vi "bt_host_rule.vi"(11 "배열":sgl[](array[numeric])) -> (2 "Received":bool=TRUE, 3 "Correct?":bool)   [LabVIEW 2023]
panel:
  out "Raw Data":sgl[](array[numeric])
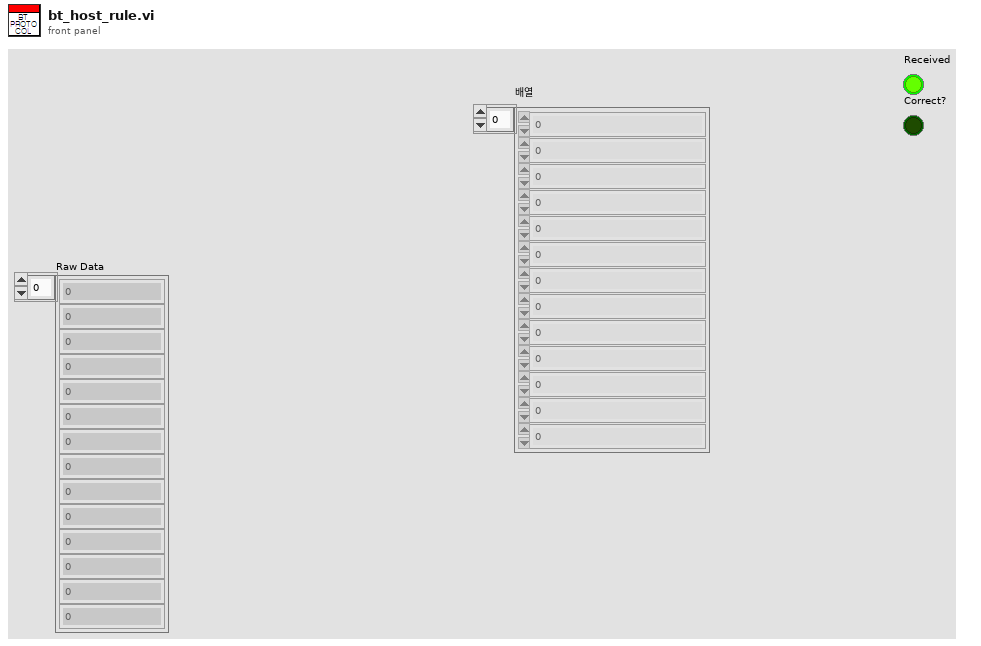
[diagram p1: front panel]
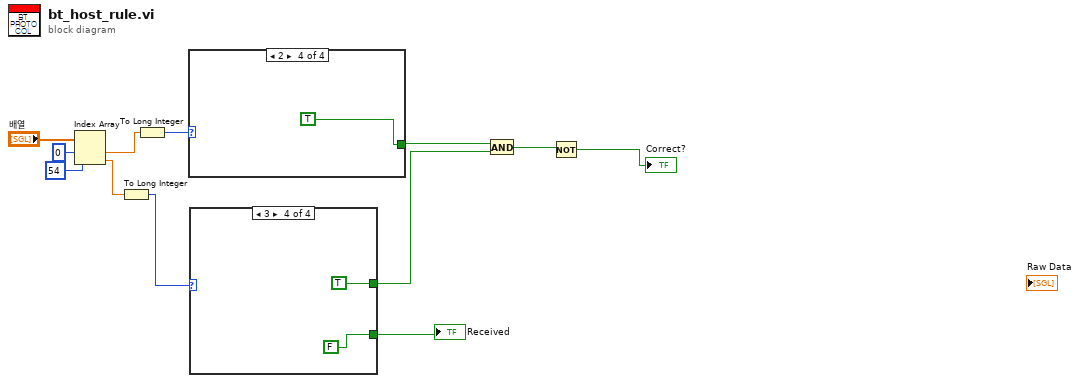
[diagram p0: block diagram]
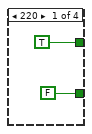
[diagram p2: hidden frame]
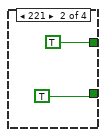
[diagram p3: hidden frame]
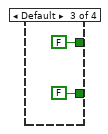
[diagram p4: hidden frame]
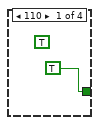
[diagram p5: hidden frame]
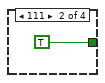
[diagram p6: hidden frame]
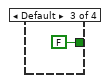
[diagram p7: hidden frame]
diagram:
  n1 = Index Array(array="배열", index #1=0 ("인덱스"), index #2=54 ("인덱스")) -> (element #1=w9:sgl, element #2=w6:sgl)
  n2 = To Long Integer(number=w6) -> (32bit integer=w5:i32)
  n3 = To Long Integer(number=w9) -> (32bit integer=w8:i32)
  n4 = case shown="2" w8 {
    tunnel: [TRUE TRUE FALSE TRUE] -> w7
    frame 110 {
      (unwired) TRUE
    }
    frame 111 {
    }
    frame Default {
    }
    frame 2 {
    }
  }
  n5 = case shown="3" w5 {
    tunnel: [TRUE TRUE FALSE TRUE] -> w4
    tunnel: [FALSE TRUE FALSE FALSE] -> w3
    frame 220 {
    }
    frame 221 {
    }
    frame Default {
    }
    frame 3 {
    }
  }
  "Received" <- w3
  n6 = And(x=w7, y=w4) -> (x .and. y?=w2:bool)
  n7 = Not(x=w2) -> (.not. x?=→"Correct?":bool)
